vi "Raft_wars_Ver4.vi"() -> ()   [LabVIEW 2026]
panel:
  out "Array":dbl[][](array[numeric])
  in  "Player Ship Inputs":T1(array[cluster]) {"Y-Coordinate" min=0 max=7; "X-Coordinate" min=0 max=7}
  in  "Emergency Stop":bool
  out "Game Status":string
  out "Ships Placed":dbl
  out "Losses":dbl
  out "Computer Hits":dbl
  out "Wins":dbl
  out "Player Hits":dbl
  in  "Attack":bool
  in  "Play Again":bool
  in  "Place Ship":bool
  in  "Attack Y":dbl
  in  "Attack X":dbl
  in  "Ship Y":i32
  in  "Ship X":i32
  out "Computer  Board":u32[][][][][][][][](array[colorbox])
  out "Player Board":u32[][][][][][][][](array[colorbox])
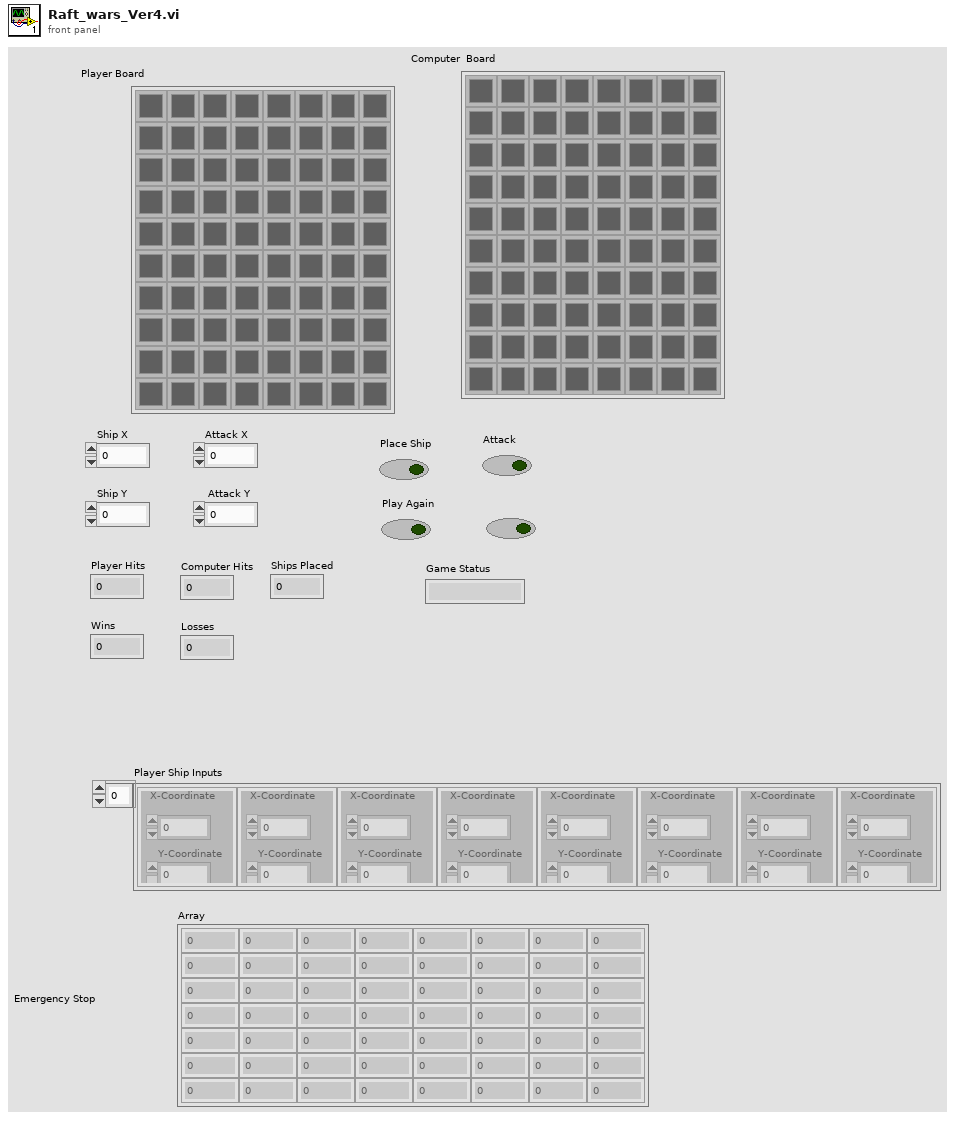
[diagram p1: front panel]
types:
  T1 = cluster{"X-Coordinate":i32, "Y-Coordinate":i32}[]
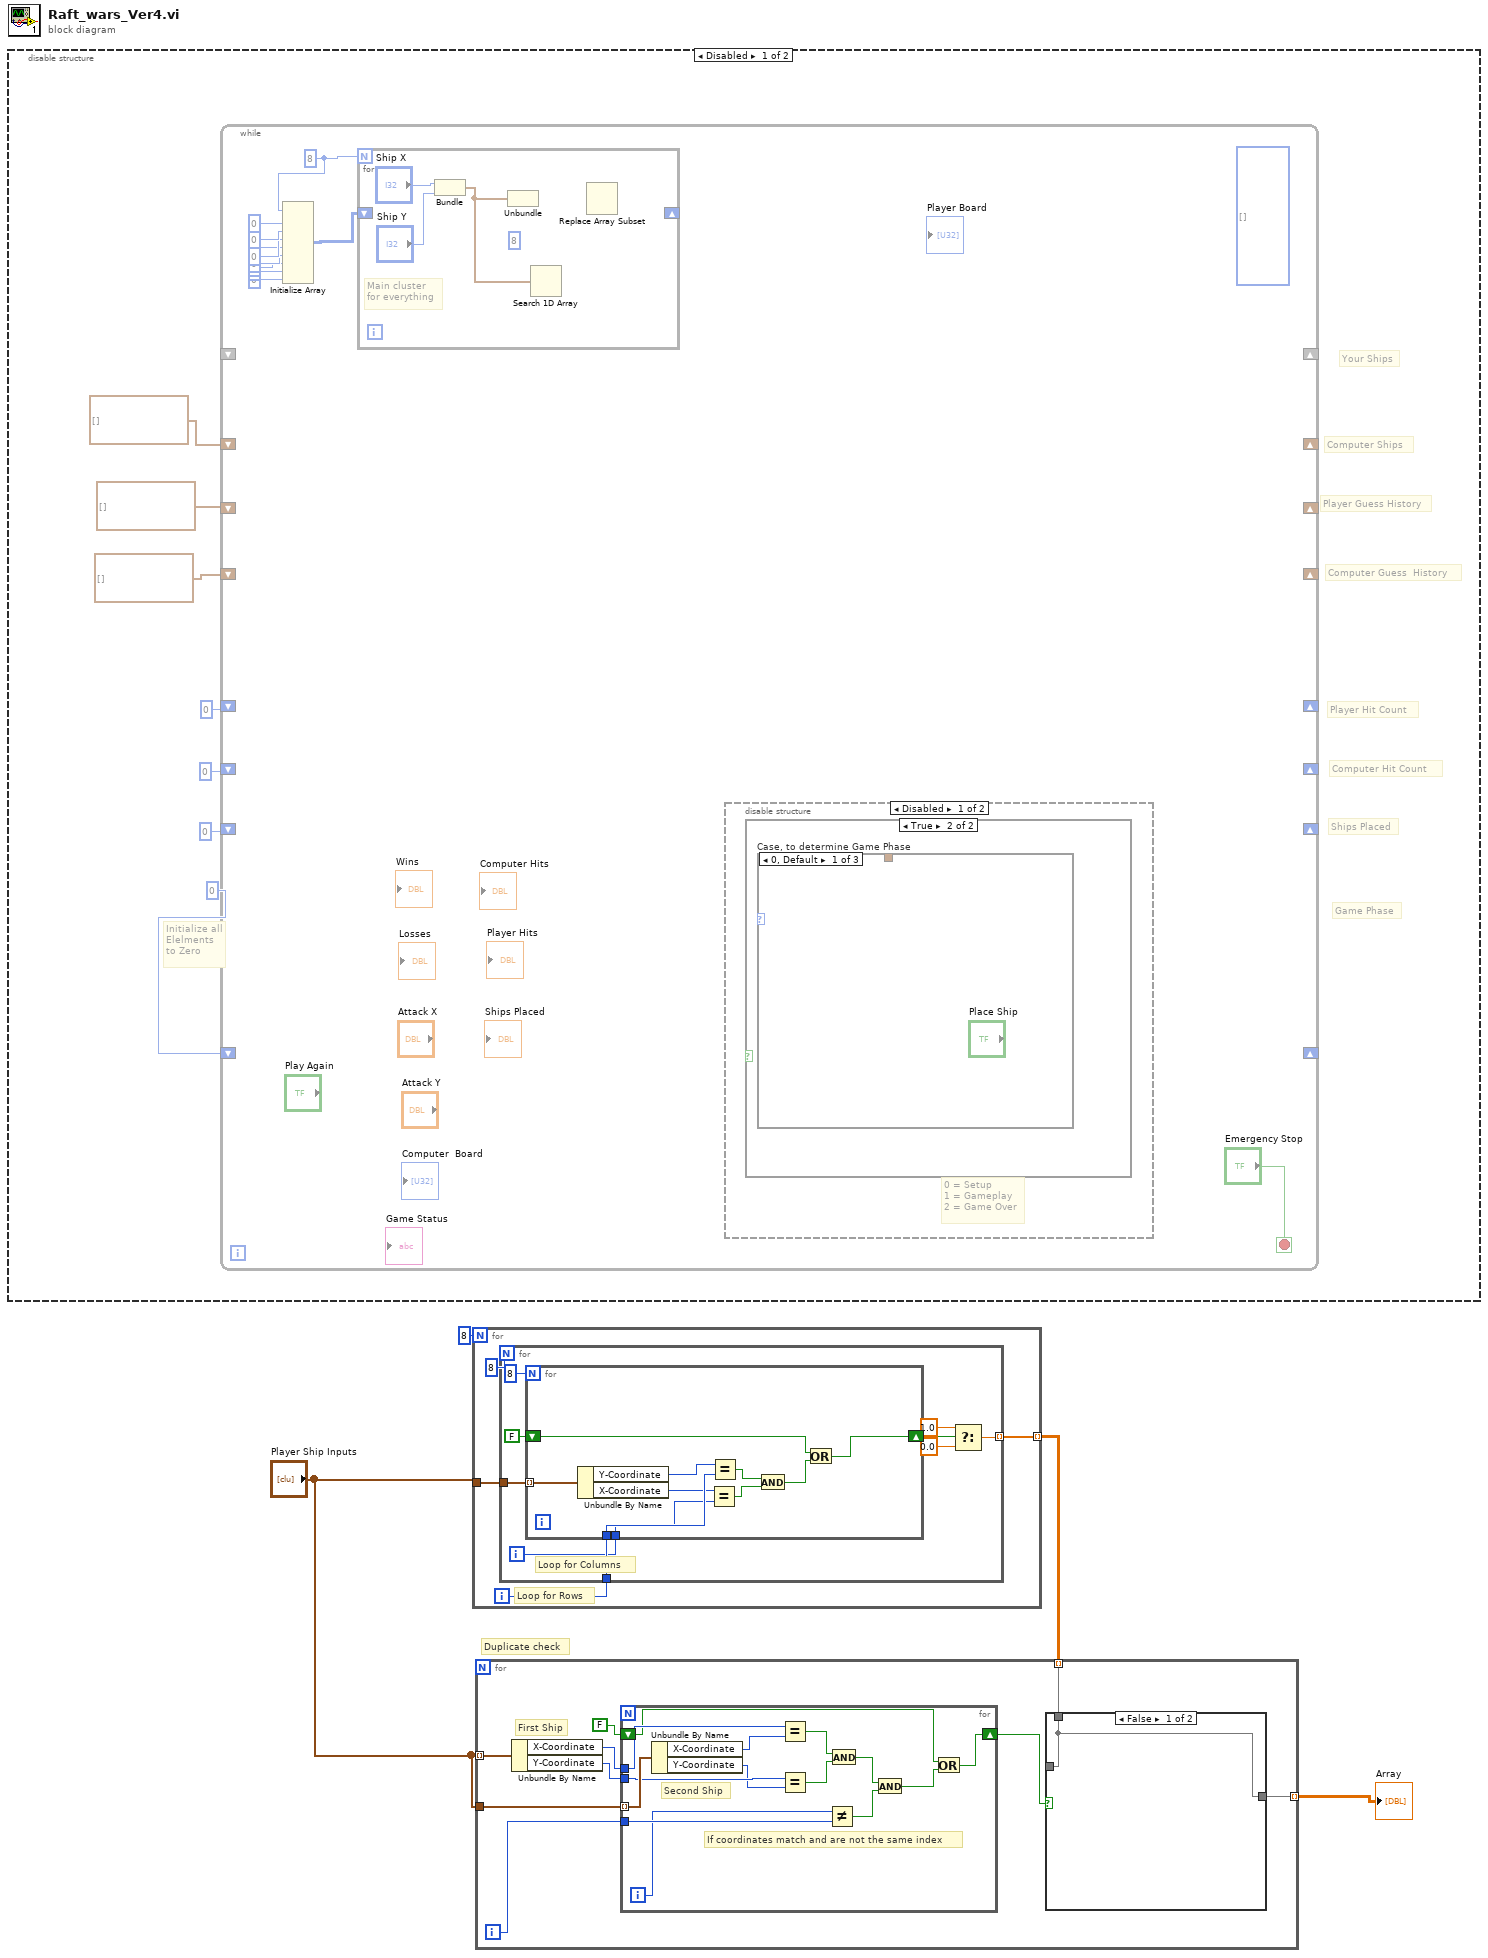
[diagram p0: block diagram]
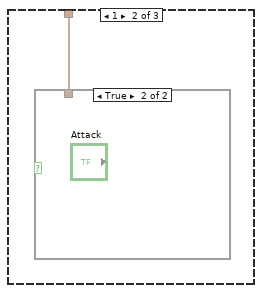
[diagram p3: hidden frame]
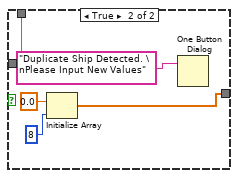
[diagram p8: hidden frame]
diagram:
  # "Duplicate check"
  n1 = disable-structure shown="Disabled" {
    frame Disabled {
      # "Initialize all\nElelments\nto Zero"
      # "Ships Placed"
      # "Your Ships"
      # "Computer Ships"
      # "Player Guess History"
      # "Computer Guess  History"
      # "Player Hit Count"
      # "Computer Hit Count"
      # "Game Phase"
      n2 = while {
        shift-right: _ -> [_]
        shift-left: _ -> [_]
        shift-right: _ -> [_]
        shift-left: cluster{dbl, dbl}[] [] -> [_]
        shift-right: _ -> [_]
        shift-left: cluster{dbl, dbl}[] [] -> [_]
        shift-right: _ -> [_]
        shift-left: cluster{dbl, dbl}[] [] -> [_]
        shift-right: _ -> [_]
        shift-left: 0 -> [_]
        shift-right: _ -> [_]
        shift-left: 0 -> [_]
        shift-right: _ -> [_]
        shift-left: 0 -> [_]
        shift-right: _ -> [_]
        shift-left: 0 -> [_]
        stop <- "Emergency Stop" stop-if-true
        w20 = 8
        (unwired) u32[][][][][][][][] [] ("PLayer 1 Board 2")
        n3 = Initialize Array(w20, 0 ("dimension size"), 0 ("dimension size"), 0 ("dimension size"), 0 ("dimension size"), 0 ("dimension size"), 0 ("dimension size"), 0 ("dimension size"), 0 ("dimension size")) -> (w21:i32[][][][][][][][])
        n4 = for {
          N: w20 -> [_]
          shift-right: _ -> [w23]
          shift-left: w21 -> [_]
          (unwired) 8
          # "Main cluster\nfor everything"
          n5 = Bundle("Ship X"="Ship X", "Ship Y"="Ship Y") -> (w24:cluster{"Ship X":i32, "Ship Y":i32})  [unwired: 1 in]
          n6 = Unbundle(w24) -> ()  [unwired: 2 out]
          n7 = Search 1D Array(element=w24) -> ()  [unwired: 2 in, 1 out]
          n8 = Replace Array Subset() -> ()  [unwired: 3 in, 1 out]
        }
        n9 = disable-structure shown="Disabled" {
          frame Disabled {
            # "0 = Setup\n1 = Gameplay\n2 = Game Over"
            n10 = case shown="True" {
              selector: _ -> [_ _]
              frame False {
              }
              frame True {
                n11 = case "Case, to determine Game Phase" shown="0, Default" {
                  selector: _ -> [_ _ _]
                  tunnel: _ -> [_ w27 _]
                  frame 0, Default {
                  }
                  frame 1 {
                    n12 = case shown="True" {
                      selector: _ -> [_ _]
                      tunnel: w27 -> [_ _]
                      frame False {
                      }
                      frame True {
                      }
                    }
                  }
                  frame 2 {
                  }
                }
              }
            }
          }
          frame Enabled {
          }
        }
      }
    }
    frame Enabled {
    }
  }
  n13 = for {
    N: 8 -> [_]
    tunnel: "Player Ship Inputs" -> [w28]
    tunnel: [w29] -> w2 mode=indexing
    i -> [w30]
    # "Loop for Rows"
    n14 = for {
      N: 8 -> [_]
      tunnel: w30 -> [w40]
      tunnel: [w35] -> w29 mode=indexing
      tunnel: w28 -> [w32]
      i -> [w39]
      # "Loop for Columns"
      n15 = for {
        N: 8 -> [_]
        tunnel: w40 -> [w44]
        tunnel: w39 -> [w43]
        shift-right: [w45] -> w38
        shift-left: FALSE -> [w46]
        tunnel: w32 -> [w42] mode=indexing
        n16 = Unbundle By Name(w42) -> ("Y-Coordinate"=w50:i32, "X-Coordinate"=w41:i32)
        n17 = Equal?(x=w41, y=w43) -> (x = y?=w48:bool)
        n18 = Equal?(x=w50, y=w44) -> (x = y?=w49:bool)
        n19 = And(x=w49, y=w48) -> (x .and. y?=w47:bool)
        n20 = Or(x=w46, y=w47) -> (x .or. y?=w45:bool)
      }
      n21 = Select(t=1.0, s=w38, f=0.0) -> (s? t:f=w35:dbl)
    }
  }
  n22 = for {
    tunnel: "Player Ship Inputs" -> [w54] mode=indexing
    tunnel: [w55] -> w3 mode=indexing
    tunnel: w2 -> [w53] mode=indexing
    tunnel: "Player Ship Inputs" -> [w52]
    i -> [w57]
    # "First Ship"
    n23 = Unbundle By Name(w54) -> ("X-Coordinate"=w59:i32, "Y-Coordinate"=w58:i32)
    n24 = for {
      tunnel: w52 -> [w79] mode=indexing
      tunnel: w59 -> [w78]
      tunnel: w58 -> [w76]
      tunnel: w57 -> [w72]
      shift-right: [w66] -> w51
      shift-left: FALSE -> [w68]
      i -> [w71]
      # "If coordinates match and are not the same index"
      # "Second Ship"
      n25 = Unbundle By Name(w79) -> ("X-Coordinate"=w77:i32, "Y-Coordinate"=w75:i32)
      n26 = Equal?(x=w78, y=w77) -> (x = y?=w73:bool)
      n27 = Equal?(x=w76, y=w75) -> (x = y?=w74:bool)
      n28 = Not Equal?(x=w71, y=w72) -> (x != y?=w69:bool)
      n29 = And(x=w73, y=w74) -> (x .and. y?=w70:bool)
      n30 = And(x=w70, y=w69) -> (x .and. y?=w67:bool)
      n31 = Or(x=w68, y=w67) -> (x .or. y?=w66:bool)
    }
    n32 = case shown="False" w51 {
      tunnel: [w60 w63] -> w55
      tunnel: [w60 w61] -> _
      tunnel: w53 -> [w60 w61]
      frame False {
      }
      frame True {
        n33 = Initialize Array(0.0 ("element"), 8 ("dimension size")) -> (w63:dbl[])
        n34 = One Button Dialog(message="Duplicate Ship Detected. \nPlease Input New Values") -> ()  [unwired: 1 in, 1 out]
      }
    }
  }
  "Array" <- w3
